vi "Read Shared Variable.vi"(11 "String":string="ni.var.psp://laserbay-dev/Logger Master/Alarms") -> (0 "error out":errorcluster, 3 "Value out":string)   [LabVIEW 2013]
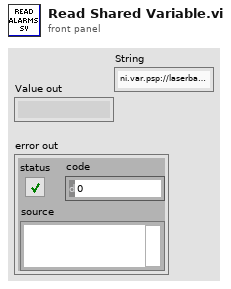
[diagram p1: front panel]
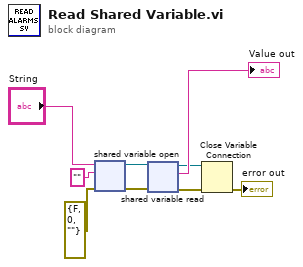
[diagram p0: block diagram]
diagram:
  n1 = shared-variable-open("String", errorcluster {"status"=FALSE, "code"=0, "source"=""} ("error in (no error)"), "") -> (w1:refnum<k21>, w2:errorcluster)  [unwired: 1 in]
  n2 = shared-variable-read(w1, w2) -> (w4:refnum<k21>, w3:errorcluster, →"Value out":string)  [unwired: 1 out]
  n3 = Close Variable Connection(8:w3, 11:w4) -> (0:→"error out":errorcluster)
